vi "Get Settings.vi"(8 "error in (no error)":errorcluster, 11 "App Settings in":refnum<class "App Settings.lvclass">) -> (0 "error out":errorcluster, 2 "Settings":T1, 3 "App Settings out":refnum<class "App Settings.lvclass">)   [LabVIEW 2017, in "Application.lvlib" / "App Settings.lvclass"]
uses:
  App Settings.lvclass
  Class Settings -- Cluster.ctl
  <vilib>/TSS/ACRObat Test Framework/Classes/Data/Data Viewer/Settings/Pass Fail Criteria -- Cluster.ctl
  App Settings.lvclass/App Settings.ctl
  <vilib>/TSS/ACRObat Test Framework/Classes/Data/Data Viewer/Settings/Data Viewer Settings.lvclass
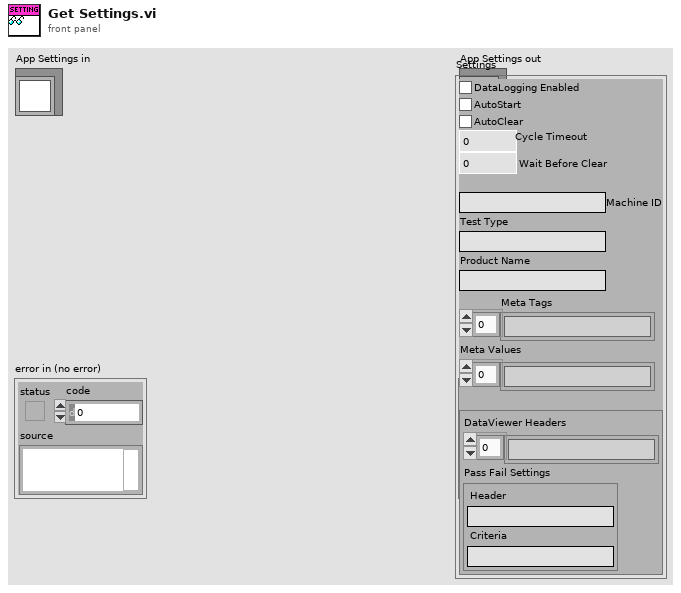
[diagram p1: front panel]
types:
  T1 = typedef "Application.lvlib/App Settings.lvclass/Class Settings -- Cluster.ctl" = cluster{"DataLogging Enabled":bool, "AutoStart":bool, "AutoClear":bool, "Cycle Timeout":u32, "Wait Before Clear":u32, "Machine ID":string, "Test Type":string, "Product Name":string, "Meta Tags":string[], "Meta Values":string[], "Viewer Settings":cluster{"DataViewer Headers":string[], "Pass Fail Settings":T2}}
  T2 = typedef "Data Viewer.lvlib/Data Viewer Settings.lvclass/Pass Fail Criteria -- Cluster.ctl" = cluster{"Header":string, "Criteria":string}
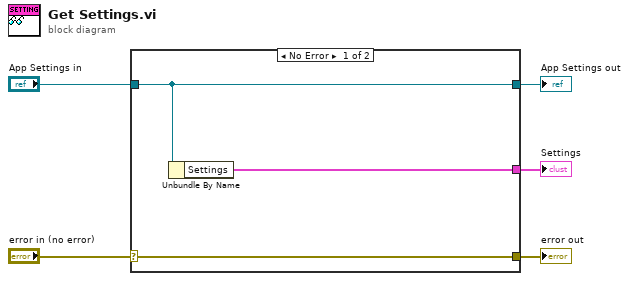
[diagram p0: block diagram]
diagram:
  n1 = case shown="No Error" "error in (no error)" {
    selector: "error in (no error)" -> [w8 w9]
    tunnel: [w8 w9] -> w4
    tunnel: [w7 w10] -> w2
    tunnel: "App Settings in" -> [w7 w10]
    tunnel: [w6 _] -> w1
    frame No Error {
      n2 = Unbundle By Name(w7) -> ("Settings"=w6:T1)
    }
    frame Error {
    }
  }
  "error out" <- w4
  "App Settings out" <- w2
  "Settings" <- w1
